vi "Teleop.vi"(10 "Match Info":T1={"Autonomous Elapsed Seconds"=0.0, "TeleOp Elapsed Seconds"=0.0, "Disabled Elapsed Seconds"=0.0, "Visited Autonomous"=FALSE, "Visited TeleOp"=FALSE, "Visited Disabled"=FALSE, "Autonomous Settings"={"Autonomous Style"=enum."Independent", "VI Refnum"=refnum}}, 11 "Call Context":T2) -> ()   [LabVIEW 2011]
doc: "This VI is called for each TeleOp packet received from the DS where the robot is not disabled. It is often used to read from the joysticks and update I/O or to update setpoints for timed control loops. It should complete and return within 20 milliseconds or it may miss DS packets."
uses:
  <vilib>/Rock Robotics/WPI/DriverStation/WPI_DriverStationDerivedRobotMode.ctl
  <vilib>/Rock Robotics/WPI/DriverStation/WPI_DriverStationMatch Info.ctl
  <vilib>/Rock Robotics/WPI/Relay/WPI_RelayValue.ctl
  Robot Global Data.vi
  System Set Points and States.vi
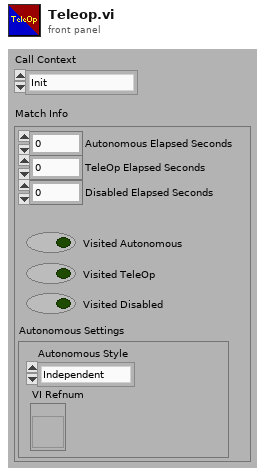
[diagram p1: front panel]
types:
  T1 = typedef "WPI_DriverStationMatch Info.ctl" = cluster{"Autonomous Elapsed Seconds":dbl, "TeleOp Elapsed Seconds":dbl, "Disabled Elapsed Seconds":dbl, "Visited Autonomous":bool, "Visited TeleOp":bool, "Visited Disabled":bool, "Autonomous Settings":cluster{"Autonomous Style":enum16{"Iterative", "Independent"}, "VI Refnum":refnum<vi>}}
  T2 = typedef "WPI_DriverStationDerivedRobotMode.ctl" = enum16{"Init", "Execute", "Stop"}
  T3 = typedef "WPI_JoystickDevRef.ctl" = cluster{"Device":T4}
  T4 = typedef "WPI_JoystickDeviceEnum.ctl" = enum16{"USB 1", "USB 2", "USB 3", "USB 4", "Kinect 1", "Kinect 2"}
  T5 = typedef "WPI_JoystickButtonState.ctl" = cluster{"Button 1":bool, "Button 2":bool, "Button 3":bool, "Button 4":bool, "Button 5":bool, "Button 6":bool, "Button 7":bool, "Button 8":bool, "Button 9":bool, "Button 10":bool, "Button 11":bool, "Button 12":bool}
  T6 = cluster{"axis 1 (x)":dbl, "axis 2 (y)":dbl, "axis 3 (throttle)":dbl, "axis 4":dbl, "axis 5":dbl, "axis 6":dbl}
  T7 = typedef "WPI_RelayDevRef.ctl" = cluster{"DevStatus":errorcluster, "Relay Channel":T8, "Digital Module":T9, "Relay Direction":T10}
  T8 = typedef "FPGA_DIORelayChannel.ctl" = enum8{"Relay 1", "Relay 2", "Relay 3", "Relay 4", "Relay 5", "Relay 6", "Relay 7", "Relay 8", "Invalid"}
  T9 = typedef "FPGA_TypedefDigitalModule.ctl" = enum16{"Digital Module 1", "Digital Module 2"}
  T10 = typedef "WPI_RelayDirection.ctl" = enum16{"Both directions", "Forward only", "Reverse only"}
  T11 = typedef "WPI_DigitalInputDevRef.ctl" = cluster{"DevStatus":errorcluster, "DIO Channel":T12, "Digital Module":T9}
  T12 = typedef "FPGA_DIOChannel.ctl" = enum8{"DIO 1", "DIO 2", "DIO 3", "DIO 4", "DIO 5", "DIO 6", "DIO 7", "DIO 8", "DIO 9", "DIO 10", "DIO 11", "DIO 12", "DIO 13", "DIO 14", "Invalid"}
  T13 = typedef "WPI_RelayValue.ctl" = enum16{"Off", "On", "Forward", "Reverse"}
  T14 = typedef "WPI_RobotDriveDevRef.ctl" = cluster{"DevStatus":errorcluster, "Motors[]":T15[], "Square Inputs":bool, "Max Output":dbl, "Isochronous":bool}
  T15 = typedef "WPI_MotorControlDeviceRef.ctl" = cluster{"DeviceStatus":errorcluster, "Type":enum16{"PWM", "CAN"}, "PWM":cluster{"Digital Module":T9, "PWM Channel":T16, "DeadBand":T17}, "CAN":cluster{"Device Number":u8, "Control Mode":T18, "Semaphore":T19, "Max Vout":dbl}, "Invert":bool, "TransformRef":T20, "InvTransformRef":T20}
  T16 = typedef "FPGA_DIOPWMChannel.ctl" = enum8{"PWM 1", "PWM 2", "PWM 3", "PWM 4", "PWM 5", "PWM 6", "PWM 7", "PWM 8", "PWM 9", "PWM 10", "Invalid"}
  T17 = typedef "WPI_PWMDeadband.ctl" = cluster{"Name":string, "maxPositivePwm":i32, "minPositivePwm":i32, "centerPwm":i32, "maxNegativePwm":i32, "minNegativePwm":i32, "angularRange":u16}
  T18 = typedef "WPI_CANJaguar_ControlMode.ctl" = enum8{"Percent VBus", "Current", "Speed", "Position", "Voltage"}
  T19 = typedef "Semaphore RefNum" = refnum<k1>
  T20 = typedef "WPI_PWMTransform_ConPane.ctl" = refnum<vi>
  T21 = typedef "WPI_AnalogChannelDevRef.ctl" = cluster{"DevStatus":errorcluster, "Analog Module":T22, "Analog Channel":T23}
  T22 = typedef "FPGA_TypedefAnalogModule.ctl" = enum16{"Analog Module 1", "Analog Module 2"}
  T23 = typedef "FPGA_AIChannel.ctl" = enum8{"AI 1", "AI 2", "AI 3", "AI 4", "AI 5", "AI 6", "AI 7", "AI 8", "Invalid"}
  T24 = cluster{"Position":cluster{"X":dbl, "Y":dbl}, "Distance (ft)":dbl}[]
  T25 = cluster{"Target Info[0]":cluster{"Position":cluster{"X":dbl, "Y":dbl}, "Distance (ft)":dbl}, "Target Info[1]":cluster{"Position":cluster{"X":dbl, "Y":dbl}, "Distance (ft)":dbl}, "Target Info[2]":cluster{"Position":cluster{"X":dbl, "Y":dbl}, "Distance (ft)":dbl}, "Target Info[3]":cluster{"Position":cluster{"X":dbl, "Y":dbl}, "Distance (ft)":dbl}, "Target Info[4]":cluster{"Position":cluster{"X":dbl, "Y":dbl}, "Distance (ft)":dbl}, "Target Info[5]":cluster{"Position":cluster{"X":dbl, "Y":dbl}, "Distance (ft)":dbl}, "Target Info[6]":cluster{"Position":cluster{"X":dbl, "Y":dbl}, "Distance (ft)":dbl}, "Target Info[7]":cluster{"Position":cluster{"X":dbl, "Y":dbl}, "Distance (ft)":dbl}, "Target Info[8]":cluster{"Position":cluster{"X":dbl, "Y":dbl}, "Distance (ft)":dbl}}
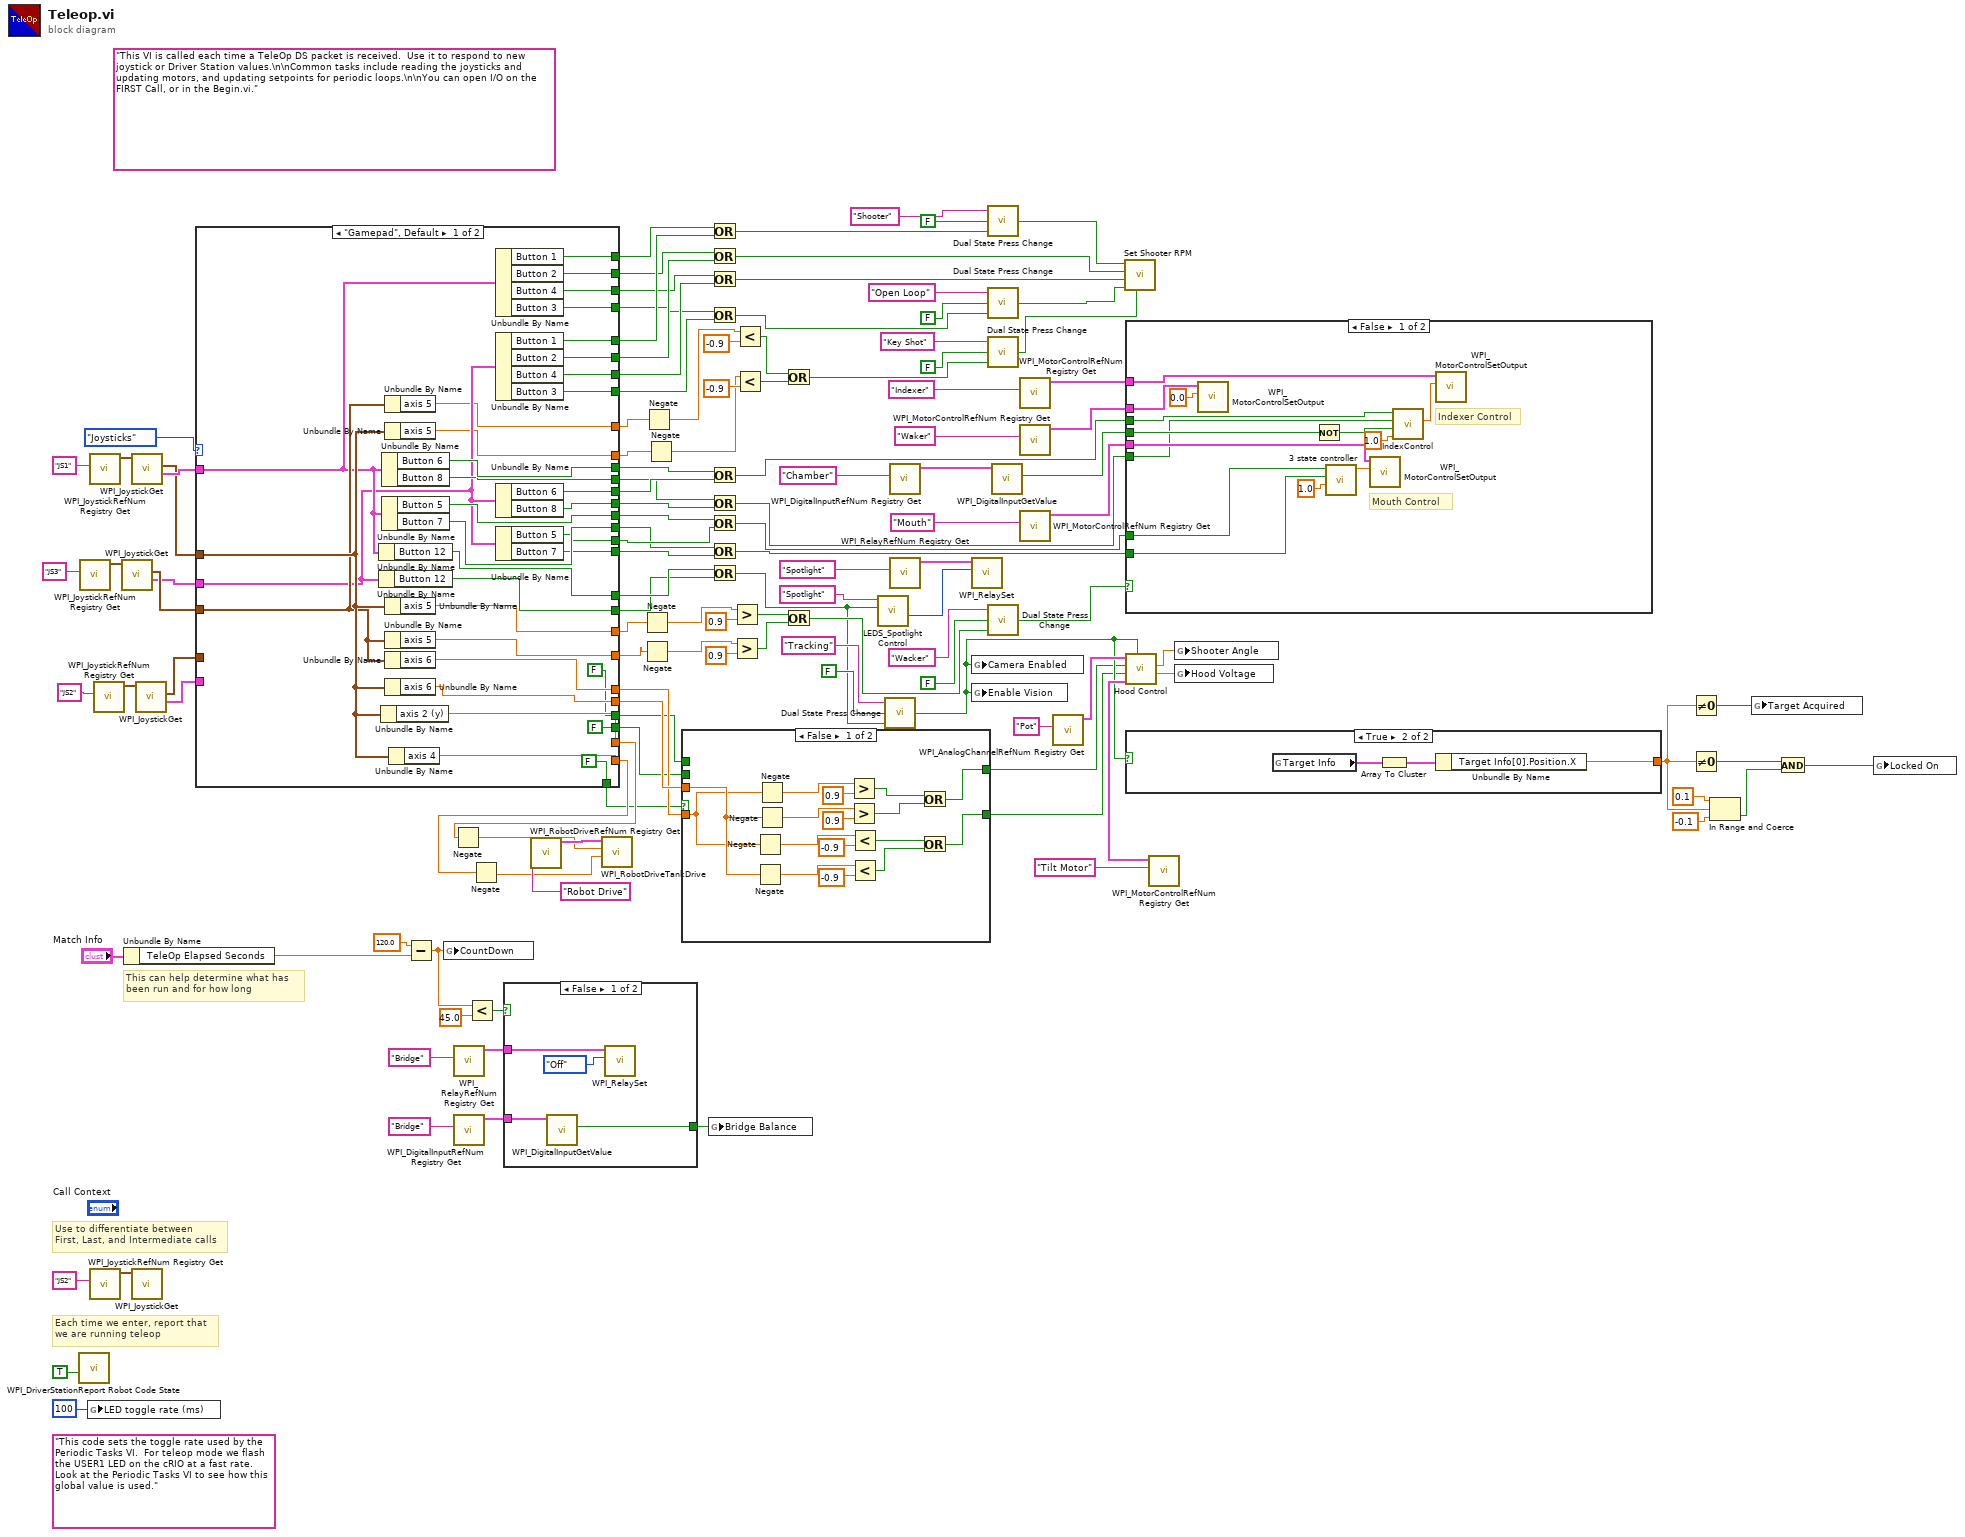
[diagram p0: block diagram]
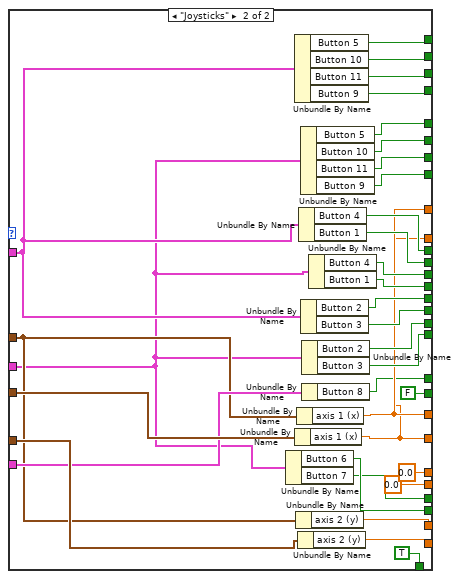
[diagram p3: hidden frame]
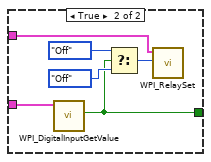
[diagram p4: hidden frame]
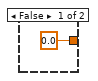
[diagram p5: hidden frame]
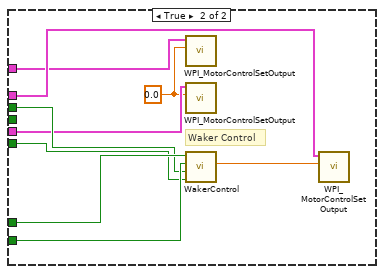
[diagram p6: hidden frame]
diagram:
  (unwired) "This code sets the toggle rate used by the Periodic Tasks VI.  For teleop mode we flash the USER1 LED on the cRIO at a fast rate.  Look at the Periodic Tasks VI to see how this global value is used."
  (unwired) "This VI is called each time a TeleOp DS packet is received.  Use it to respond to new joystick or Driver Station values.\n\nCommon tasks include reading the joysticks and updating motors, and updating setpoints for periodic loops.\n\nYou can open I/O on the FIRST Call, or in the Begin.vi."
  # "Each time we enter, report that\nwe are running teleop"
  # "Use to differentiate between\nFirst, Last, and Intermediate calls"
  # "This can help determine what has\nbeen run and for how long"
  n1 = call <vilib>:"WPI_DriverStationReport Robot Code State.vi"("TeleOp"=TRUE ("Autonomous")) -> ()  [unwired: 10 in, 1 out]
  n2 = call <vilib>:"WPI_JoystickRefNum Registry Get.vi"("refnum name"="JS3") -> ("JoystickDevRef"=w23:T3)  [unwired: 9 in, 1 out]
  n3 = global write "Robot Global Data.vi" "LED toggle rate (ms)"(u32 100 ("LED ms toggle rate")) -> ()
  n4 = call <vilib>:"WPI_JoystickRefNum Registry Get.vi"("refnum name"="JS1") -> ("JoystickDevRef"=w123:T3)  [unwired: 9 in, 1 out]
  n5 = call <vilib>:"WPI_JoystickRefNum Registry Get.vi"("refnum name"="JS2") -> ("JoystickDevRef"=w76:T3)  [unwired: 9 in, 1 out]
  n6 = call <vilib>:"WPI_JoystickRefNum Registry Get.vi"("refnum name"="JS2") -> ("JoystickDevRef"=w18:T3)  [unwired: 9 in, 1 out]
  n7 = call <vilib>:"WPI_JoystickGet.vi"("JoystickDevRef"=w23) -> ("Buttons"=w21:T5, "Axes"=w22:T6)  [unwired: 4 in, 1 out]
  n8 = Unbundle By Name("Match Info") -> ("TeleOp Elapsed Seconds"=w87:dbl)
  n9 = call <vilib>:"WPI_JoystickGet.vi"("JoystickDevRef"=w123) -> ("Buttons"=w101:T5, "Axes"=w37:T6)  [unwired: 4 in, 1 out]
  n10 = call <vilib>:"WPI_JoystickGet.vi"("JoystickDevRef"=w76) -> ()  [unwired: 4 in, 3 out]
  n11 = call <vilib>:"WPI_JoystickGet.vi"("JoystickDevRef"=w18) -> ("Buttons"=w16:T5, "Axes"=w17:T6)  [unwired: 4 in, 1 out]
  n12 = case shown="\"Gamepad\", Default" enum16{"Gamepad", "Joysticks"}."Joysticks" {
    tunnel: [w138 w173] -> w11
    tunnel: w101 -> [w140 w178]
    tunnel: [w135 0.0 ("axis 6")] -> w83
    tunnel: [w152 w190] -> w75
    tunnel: [w151 w186] -> w74
    tunnel: [w150 w189] -> w72
    tunnel: [w149 w185] -> w71
    tunnel: [w145 w184] -> w69
    tunnel: [w148 w187] -> w68
    tunnel: [w146 w183] -> w66
    tunnel: [w147 w188] -> w65
    tunnel: [w159 w177] -> w63
    tunnel: [w160 w182] -> w62
    tunnel: [w157 w181] -> w60
    tunnel: [w158 w176] -> w59
    tunnel: [w156 w180] -> w57
    tunnel: [w154 w175] -> w56
    tunnel: [w155 w179] -> w54
    tunnel: [w153 w174] -> w53
    tunnel: [w137 w172] -> w9
    tunnel: [w144 w166] -> w47
    tunnel: [w143 FALSE ("Button 12")] -> w46
    tunnel: [w136 0.0 ("axis 6")] -> w44
    tunnel: [w132 w173] -> w13
    tunnel: [w131 w172] -> w15
    tunnel: w37 -> [w142 w165]
    tunnel: w22 -> [w141 w171]
    tunnel: w21 -> [w139 w161]
    tunnel: [w133 w192] -> w5
    tunnel: [w134 w193] -> w7
    tunnel: w17 -> [_ w191]
    tunnel: w16 -> [_ w167]
    tunnel: [FALSE TRUE] -> w3
    tunnel: [FALSE ("Button 6") w164] -> w2
    tunnel: [FALSE ("Button 7") w163] -> w1
    frame "Gamepad", Default {
      n13 = Unbundle By Name(w140) -> ("Button 12"=w144:bool)
      n14 = Unbundle By Name(w139) -> ("Button 12"=w143:bool)
      n15 = Unbundle By Name(w142) -> ("axis 2 (y)"=w134:dbl)
      n16 = Unbundle By Name(w140) -> ("Button 6"=w160:bool, "Button 8"=w157:bool)
      n17 = Unbundle By Name(w140) -> ("Button 5"=w156:bool, "Button 7"=w155:bool)
      n18 = Unbundle By Name(w141) -> ("axis 5"=w132:dbl)
      n19 = Unbundle By Name(w142) -> ("axis 5"=w131:dbl)
      n20 = Unbundle By Name(w142) -> ("axis 5"=w138:dbl)
      n21 = Unbundle By Name(w141) -> ("axis 5"=w137:dbl)
      n22 = Unbundle By Name(w141) -> ("axis 6"=w136:dbl)
      n23 = Unbundle By Name(w142) -> ("axis 6"=w135:dbl)
      n24 = Unbundle By Name(w142) -> ("axis 4"=w133:dbl)
      n25 = Unbundle By Name(w140) -> ("Button 1"=w152:bool, "Button 2"=w150:bool, "Button 4"=w148:bool, "Button 3"=w147:bool)
      n26 = Unbundle By Name(w139) -> ("Button 1"=w151:bool, "Button 2"=w149:bool, "Button 4"=w145:bool, "Button 3"=w146:bool)
      n27 = Unbundle By Name(w139) -> ("Button 6"=w159:bool, "Button 8"=w158:bool)
      n28 = Unbundle By Name(w139) -> ("Button 5"=w154:bool, "Button 7"=w153:bool)
    }
    frame "Joysticks" {
      n29 = Unbundle By Name(w161) -> ("Button 6"=w164:bool, "Button 7"=w163:bool)
      n30 = Unbundle By Name(w178) -> ("Button 5"=w190:bool, "Button 10"=w189:bool, "Button 11"=w187:bool, "Button 9"=w188:bool)
      n31 = Unbundle By Name(w171) -> ("axis 1 (x)"=w172:dbl)
      n32 = Unbundle By Name(w165) -> ("axis 2 (y)"=w193:dbl)
      n33 = Unbundle By Name(w165) -> ("axis 1 (x)"=w173:dbl)
      n34 = Unbundle By Name(w191) -> ("axis 2 (y)"=w192:dbl)
      n35 = Unbundle By Name(w178) -> ("Button 4"=w182:bool, "Button 1"=w181:bool)
      n36 = Unbundle By Name(w161) -> ("Button 5"=w186:bool, "Button 10"=w185:bool, "Button 11"=w184:bool, "Button 9"=w183:bool)
      n37 = Unbundle By Name(w178) -> ("Button 2"=w180:bool, "Button 3"=w179:bool)
      n38 = Unbundle By Name(w161) -> ("Button 2"=w175:bool, "Button 3"=w174:bool)
      n39 = Unbundle By Name(w167) -> ("Button 8"=w166:bool)
      n40 = Unbundle By Name(w161) -> ("Button 4"=w177:bool, "Button 1"=w176:bool)
    }
  }
  n41 = Subtract(x=120.0, y=w87) -> (x-y=w29:dbl)
  n42 = global write "System Set Points and States.vi" "CountDown"(w29) -> ()
  n43 = Negate(x=w7) -> (-x=w6:dbl)
  n44 = call <vilib>:"WPI_RelayRefNum Registry Get.vi"("refnum name"="Bridge") -> ("RelayDevRef"=w27:T7)  [unwired: 9 in, 1 out]
  n45 = call <vilib>:"WPI_DigitalInputRefNum Registry Get.vi"("refnum name"="Bridge") -> ("DigitalInputDevRef"=w32:T11)  [unwired: 9 in, 1 out]
  n46 = Less?(x=w29, y=45.0) -> (x < y?=w30:bool)
  n47 = Negate(x=w5) -> (-x=w4:dbl)
  n48 = case shown="False" w30 {
    tunnel: w32 -> [w195 w203]
    tunnel: w27 -> [w197 w199]
    tunnel: [w194 w198] -> w25
    frame False {
      n49 = call <vilib>:"WPI_DigitalInputGetValue.vi"("DigitalInputDevRef"=w195) -> ("Value"=w194:bool)  [unwired: 8 in, 2 out]
      n50 = call <vilib>:"WPI_RelaySet.vi"("RelayValue"=WPI_RelayValue."Off", "RelayDevRef"=w197) -> ()  [unwired: 8 in, 2 out]
    }
    frame True {
      n51 = call <vilib>:"WPI_DigitalInputGetValue.vi"("DigitalInputDevRef"=w203) -> ("Value"=w198:bool)  [unwired: 8 in, 2 out]
      n52 = Select(t=WPI_RelayValue."Off" ("Relay State"), s=w198, f=WPI_RelayValue."Off" ("Relay State")) -> (s? t:f=w202:T13)
      n53 = call <vilib>:"WPI_RelaySet.vi"("RelayValue"=w202, "RelayDevRef"=w199) -> ()  [unwired: 8 in, 2 out]
    }
  }
  n54 = call <vilib>:"WPI_RobotDriveRefNum Registry Get.vi"("refnum name"="Robot Drive") -> ("RobotDriveDevRef"=w121:T14)  [unwired: 9 in, 1 out]
  n55 = call <vilib>:"WPI_RobotDriveTankDrive.vi"("Right axis value"=w4, "Left axis value"=w6, "RobotDriveDevRef"=w121) -> ()  [unwired: 7 in, 2 out]
  n56 = Negate(x=w11) -> (-x=w10:dbl)
  n57 = Negate(x=w9) -> (-x=w8:dbl)
  n58 = Negate(x=w13) -> (-x=w12:dbl)
  n59 = Negate(x=w15) -> (-x=w14:dbl)
  n60 = case shown="False" w3 {
    tunnel: w83 -> [w215 _]
    tunnel: w44 -> [w210 _]
    tunnel: [w205 w221] -> w43
    tunnel: [w204 w220] -> w42
    tunnel: w2 -> [_ w221]
    tunnel: w1 -> [_ w220]
    frame False {
      n61 = Negate(x=w210) -> (-x=w213:dbl)
      n62 = Negate(x=w215) -> (-x=w218:dbl)
      n63 = Negate(x=w210) -> (-x=w211:dbl)
      n64 = Negate(x=w215) -> (-x=w216:dbl)
      n65 = Greater?(x=w211, y=0.9) -> (0:w209:bool)
      n66 = Greater?(x=w216, y=0.9) -> (0:w208:bool)
      n67 = Less?(x=w213, y=-0.9) -> (x < y?=w207:bool)
      n68 = Less?(x=w218, y=-0.9) -> (x < y?=w206:bool)
      n69 = Or(x=w209, y=w208) -> (x .or. y?=w205:bool)
      n70 = Or(x=w207, y=w206) -> (x .or. y?=w204:bool)
    }
    frame True {
    }
  }
  n71 = global write "System Set Points and States.vi" "Bridge Balance"(w25) -> ()
  n72 = Or(x=w75, y=w74) -> (x .or. y?=w73:bool)
  n73 = Or(x=w72, y=w71) -> (x .or. y?=w70:bool)
  n74 = Or(x=w68, y=w69) -> (x .or. y?=w67:bool)
  n75 = Or(x=w65, y=w66) -> (x .or. y?=w64:bool)
  n76 = Or(x=w62, y=w63) -> (x .or. y?=w61:bool)
  n77 = Or(x=w60, y=w59) -> (x .or. y?=w58:bool)
  n78 = Or(x=w57, y=w56) -> (x .or. y?=w55:bool)
  n79 = Or(x=w54, y=w53) -> (x .or. y?=w52:bool)
  n80 = Or(x=w47, y=w46) -> (x .or. y?=w45:bool)
  n81 = Greater?(x=w10, y=0.9) -> (0:w49:bool)
  n82 = Greater?(x=w8, y=0.9) -> (0:w50:bool)
  n83 = Less?(x=w12, y=-0.9) -> (x < y?=w36:bool)
  n84 = Less?(x=w14, y=-0.9) -> (x < y?=w35:bool)
  n85 = Or(x=w36, y=w35) -> (x .or. y?=w34:bool)
  n86 = Or(x=w49, y=w50) -> (x .or. y?=w48:bool)
  n87 = call "LEDS_Spotlight Control.vi"("Name"="Spotlight", "Button"=w45) -> ("Relay State"=w96:T13)  [unwired: 8 in]
  n88 = call "Dual State Press Change.vi"("Enable/Disable"=w45, "Initial"=FALSE, "Value Name"="Tracking") -> ("Enabled"=w80:bool)
  n89 = call <vilib>:"WPI_DigitalInputRefNum Registry Get.vi"("refnum name"="Chamber") -> ("DigitalInputDevRef"=w110:T11)  [unwired: 9 in, 1 out]
  n90 = call <vilib>:"WPI_RelayRefNum Registry Get.vi"("refnum name"="Spotlight") -> ("RelayDevRef"=w98:T7)  [unwired: 9 in, 1 out]
  n91 = call <vilib>:"WPI_RelaySet.vi"("RelayValue"=w96, "RelayDevRef"=w98) -> ()  [unwired: 8 in, 2 out]
  n92 = global write "System Set Points and States.vi" "Camera Enabled"(w80) -> ()
  n93 = global write "Robot Global Data.vi" "Enable Vision"(w80) -> ()
  n94 = call "Dual State Press Change.vi"("Enable/Disable"=w73, "Initial"=FALSE, "Value Name"="Shooter") -> ("Enabled"=w102:bool)
  n95 = call "Dual State Press Change.vi"("Enable/Disable"=w64, "Initial"=FALSE, "Value Name"="Open Loop") -> ("Enabled"=w103:bool)
  n96 = call "Dual State Press Change.vi"("Enable/Disable"=w34, "Initial"=FALSE, "Value Name"="Key Shot") -> ("Enabled"=w33:bool)
  n97 = call "Dual State Press Change.vi"("Enable/Disable"=w48, "Initial"=FALSE, "Value Name"="Wacker") -> ("Enabled"=w116:bool)
  n98 = call <vilib>:"WPI_DigitalInputGetValue.vi"("DigitalInputDevRef"=w110) -> ("Value"=w108:bool)  [unwired: 8 in, 2 out]
  n99 = call <vilib>:"WPI_MotorControlRefNum Registry Get.vi"("refnum name"="Indexer") -> ("MotorControlDevRef"=w111:T15)  [unwired: 9 in, 1 out]
  n100 = call <vilib>:"WPI_MotorControlRefNum Registry Get.vi"("refnum name"="Waker") -> ("MotorControlDevRef"=w113:T15)  [unwired: 9 in, 1 out]
  n101 = call <vilib>:"WPI_MotorControlRefNum Registry Get.vi"("refnum name"="Mouth") -> ("MotorControlDevRef"=w117:T15)  [unwired: 9 in, 1 out]
  n102 = call <vilib>:"WPI_AnalogChannelRefNum Registry Get.vi"("refnum name"="Pot") -> ("AIDeviceRef"=w81:T21)  [unwired: 9 in, 1 out]
  n103 = call "Set Shooter RPM.vi"("Key Shot"=w33, "Open Loop"=w103, "Increment"=w67, "Decrement"=w70, "Shooter Enabled"=w102) -> ()  [unwired: 7 in]
  n104 = case shown="False" w116 {
    tunnel: w55 -> [w231 w243]
    tunnel: w52 -> [w230 w242]
    tunnel: w61 -> [w223 w241]
    tunnel: w58 -> [w222 w240]
    tunnel: w117 -> [w229 w237]
    tunnel: w111 -> [w228 w238]
    tunnel: w113 -> [w227 w239]
    tunnel: w108 -> [w225 _]
    frame False {
      # "Indexer Control"
      # "Mouth Control"
      n105 = call <vilib>:"WPI_MotorControlSetOutput.vi"("Output"=0.0, "MotorControlDevRef"=w227) -> ()  [unwired: 8 in, 2 out]
      n106 = Not(x=w225) -> (.not. x?=w224:bool)
      n107 = call "3 state controller.vi"("Power"=1.0, "Backward"=w230, "Forward"=w231) -> ("Numeric"=w235:dbl)  [unwired: 8 in]
      n108 = call <vilib>:"WPI_MotorControlSetOutput.vi"("Output"=w235, "MotorControlDevRef"=w229) -> ()  [unwired: 8 in, 2 out]
      n109 = call "IndexControl.vi"("Power"=1.0, "Chamber"=w224, "Back"=w222, "Forward"=w223) -> ("Numeric"=w233:dbl)  [unwired: 7 in]
      n110 = call <vilib>:"WPI_MotorControlSetOutput.vi"("Output"=w233, "MotorControlDevRef"=w228) -> ()  [unwired: 8 in, 2 out]
    }
    frame True {
      w236 = 0.0 ("Output")
      # "Waker Control"
      n111 = call <vilib>:"WPI_MotorControlSetOutput.vi"("Output"=w236, "MotorControlDevRef"=w238) -> ()  [unwired: 8 in, 2 out]
      n112 = call <vilib>:"WPI_MotorControlSetOutput.vi"("Output"=w236, "MotorControlDevRef"=w237) -> ()  [unwired: 8 in, 2 out]
      n113 = call "WakerControl.vi"("Button 4"=w240, "Button 2"=w241, "Button 3"=w242, "Button 1"=w243) -> ("Speed Out"=w244:dbl)  [unwired: 5 in]
      n114 = call <vilib>:"WPI_MotorControlSetOutput.vi"("Output"=w244, "MotorControlDevRef"=w239) -> ()  [unwired: 8 in, 2 out]
    }
  }
  n115 = case shown="True" w80 {
    tunnel: [0.0 ("Distance (ft)") w246] -> w88
    frame False {
    }
    frame True {
      n116 = global read "Robot Global Data.vi" "Target Info"() -> (w248:T24)
      n117 = Array To Cluster(array=w248) -> (cluster=w247:T25)
      n118 = Unbundle By Name(w247) -> ("Target Info[0].Position.X"=w246:dbl)
    }
  }
  n119 = call <vilib>:"WPI_MotorControlRefNum Registry Get.vi"("refnum name"="Tilt Motor") -> ("MotorControlDevRef"=w82:T15)  [unwired: 9 in, 1 out]
  n120 = call "Hood Control.vi"("Vision"=w80, "MotorControlDevRef"=w82, "Down"=w42, "Up"=w43, "AIDeviceRef"=w81) -> ("Voltage"=w78:dbl, "Shoter Angle"=w79:dbl)  [unwired: 5 in]
  n121 = global write "System Set Points and States.vi" "Shooter Angle"(w79) -> ()
  n122 = global write "System Set Points and States.vi" "Hood Voltage"(w78) -> ()
  n123 = Not Equal To 0?(x=w88) -> (x != 0?=w92:bool)
  n124 = Not Equal To 0?(x=w88) -> (x != 0?=w91:bool)
  n125 = In Range and Coerce(upper limit=0.1, x=w88, lower limit=-0.1) -> (In Range?=w90:bool)  [unwired: 1 out]
  n126 = global write "System Set Points and States.vi" "Target Acquired"(w92) -> ()
  n127 = And(x=w91, y=w90) -> (x .and. y?=w89:bool)
  n128 = global write "System Set Points and States.vi" "Locked On"(w89) -> ()
